vi "GDSII_Parser_Prototype.vi"() -> ()   [LabVIEW 2019]
uses:
  2b7293ed-e710-4ec8-a3ce-adb50af5e69b.vi
  1c682564-4fc3-4e5f-8e88-aad9faa58424.vi
  0011f8b4-c6ad-40f6-b327-4618c1387816.vi
  5f04ecbc-5114-4225-9cf0-5074f08f4171.vi
  <vilib>/JDP Science/JSONtext/Variant to JSON Text.vi
  <vilib>/JDP Science/JSONtext/LVClass Serializer/JSONtext LVClass Serializer.lvclass
panel:
  in  "Path":path=path "C:/Users/Albro/Downloads/Aditi_GDSII/Aditi_GDSII.gds"
  out "Record Str":string
  out "Record Values":string[](array[string])
  out "Record Types Array":string[](array[string])
  # "[\n    2021,\n    1,\n    24,\n    20,\n    0,\n    15,\n    2021,\n    1,\n    24,\n    20,\n    0,\n    15\n]"
  # "[\n    8.16583633422852E-9,\n    7.98085213557943E-33\n]"
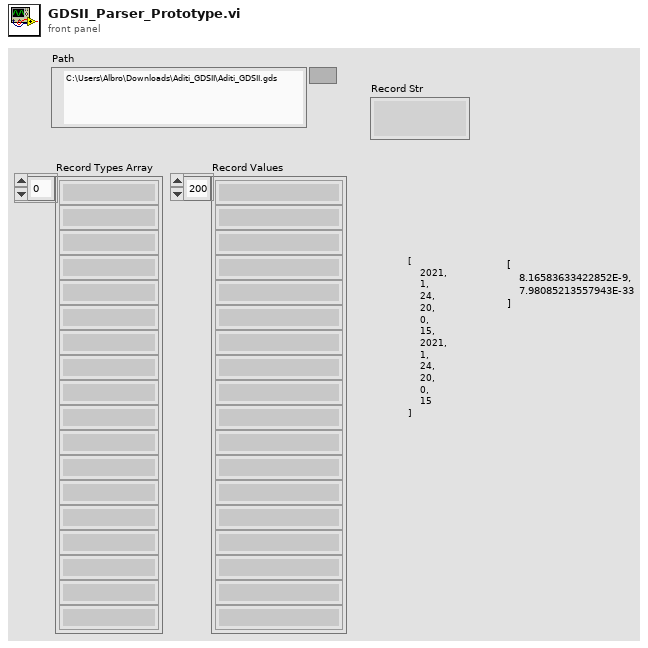
[diagram p1: front panel]
types:
  T1 = enum32{"Invalid", "Standard", "Closed", "Hidden", "Minimized", "Maximized"}
  T2 = enum32{"invalid app kind", "Development System", "Run Time System", "Student Edition", "Embedded LabVIEW", "Evaluation", "Custom"}
  T3 = cluster{"Core":cluster{"Current VI Reference":refnum<vi>, "Close Panel on Exit?":bool}, "Raw Str":string, "Record Str":string, "Records":string[], "Record Index":i32, "Record Type":i16, "Record Types Array":string[], "Record Values":string[]}
  T4 = cluster{"Current VI Reference":refnum<vi>, "Close Panel on Exit?":bool}
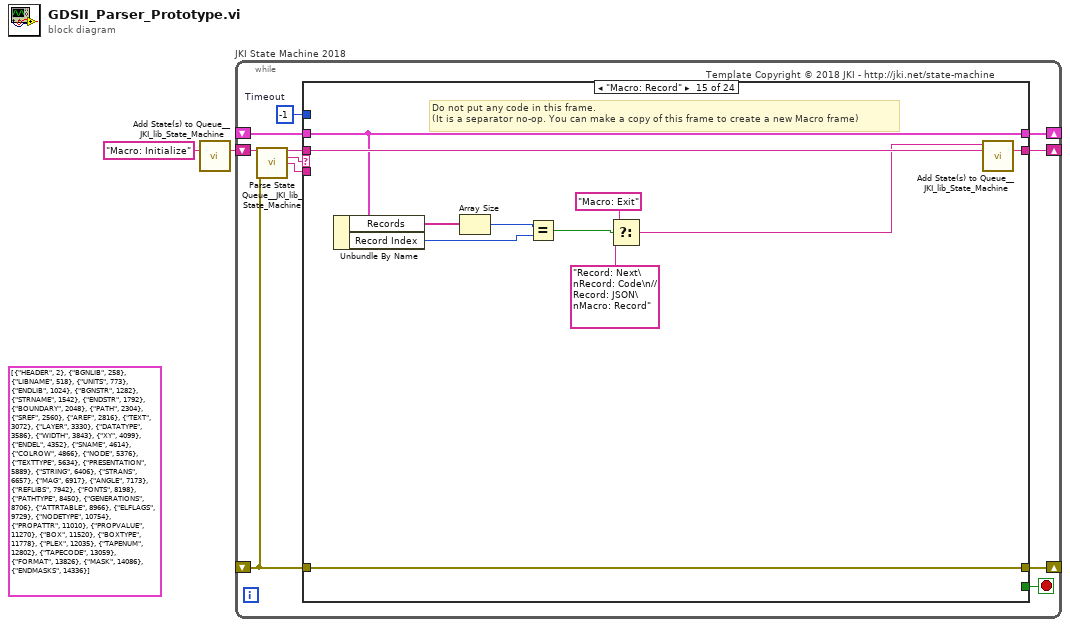
[diagram p0: block diagram]
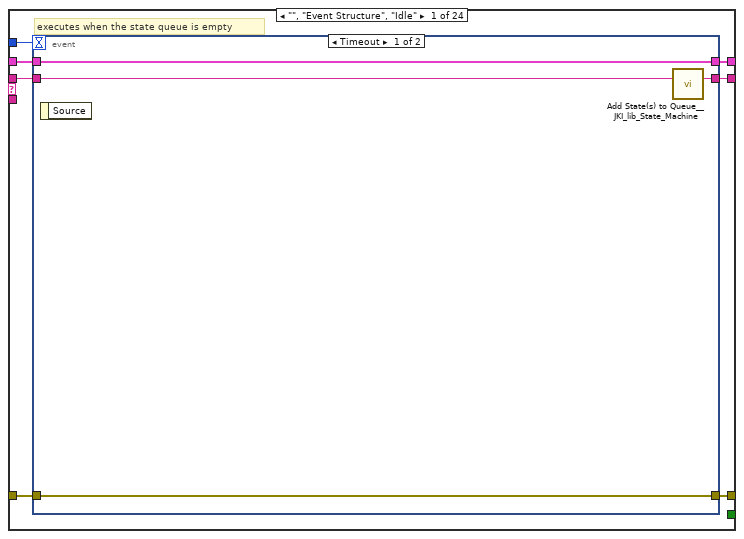
[diagram p2: hidden frame]
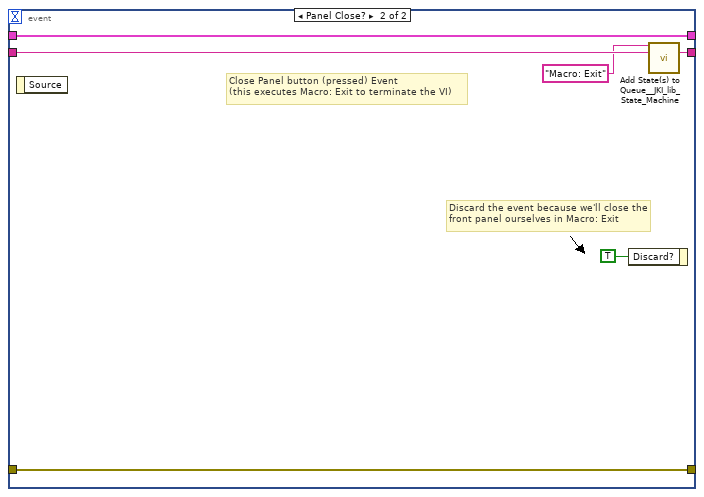
[diagram p3: hidden frame]
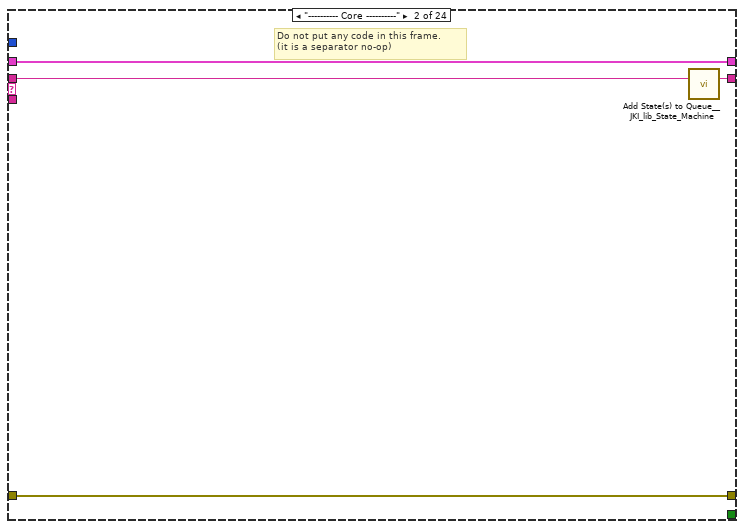
[diagram p4: hidden frame]
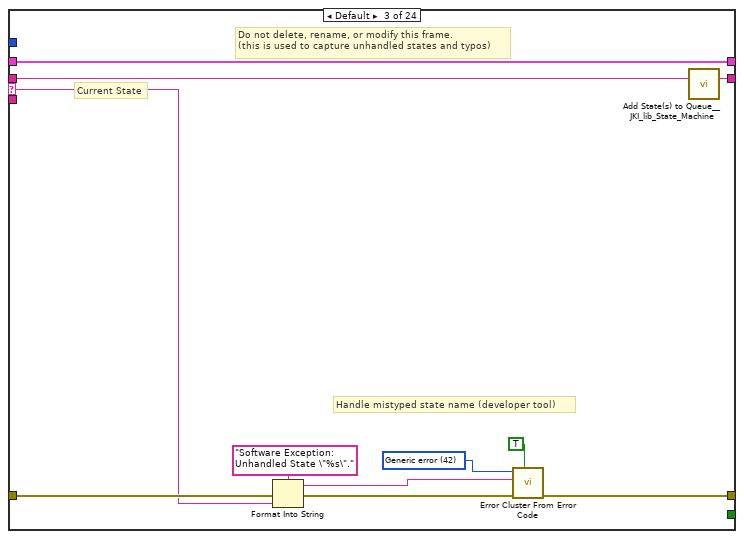
[diagram p5: hidden frame]
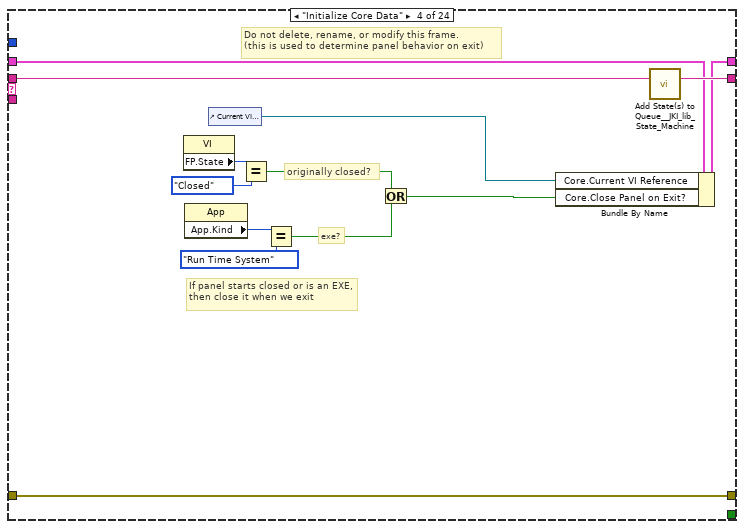
[diagram p6: hidden frame]
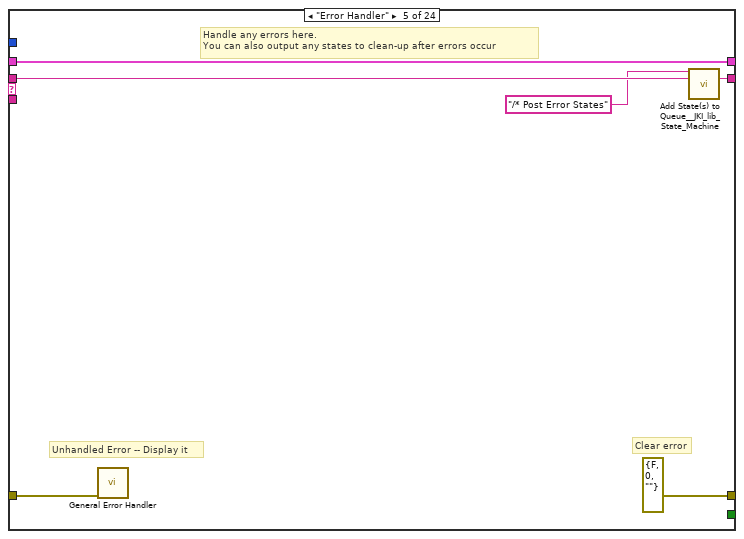
[diagram p7: hidden frame]
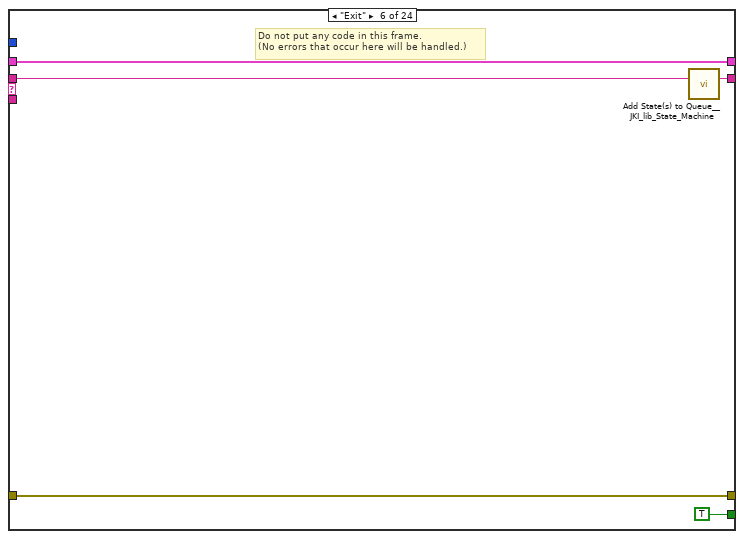
[diagram p8: hidden frame]
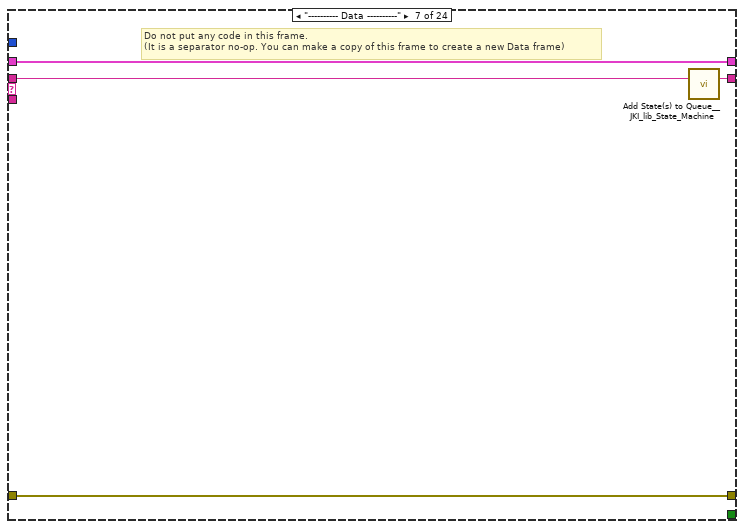
[diagram p9: hidden frame]
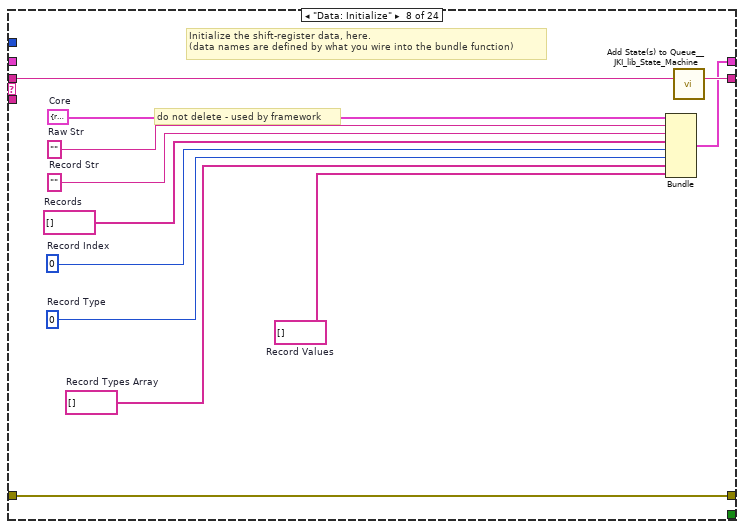
[diagram p10: hidden frame]
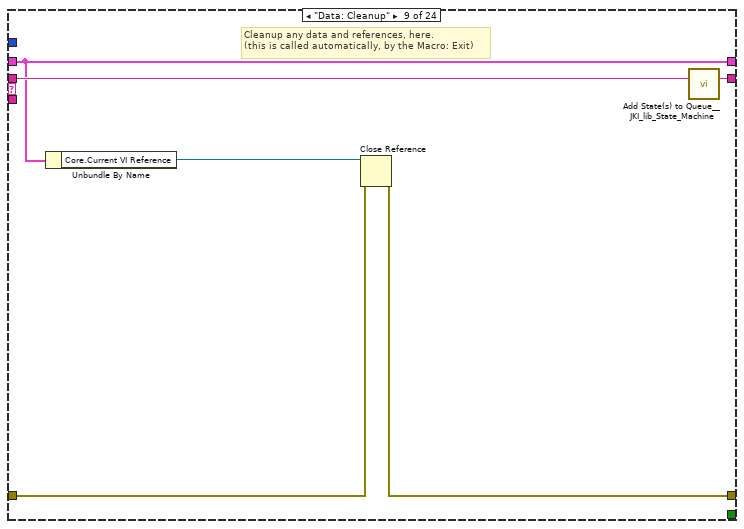
[diagram p11: hidden frame]
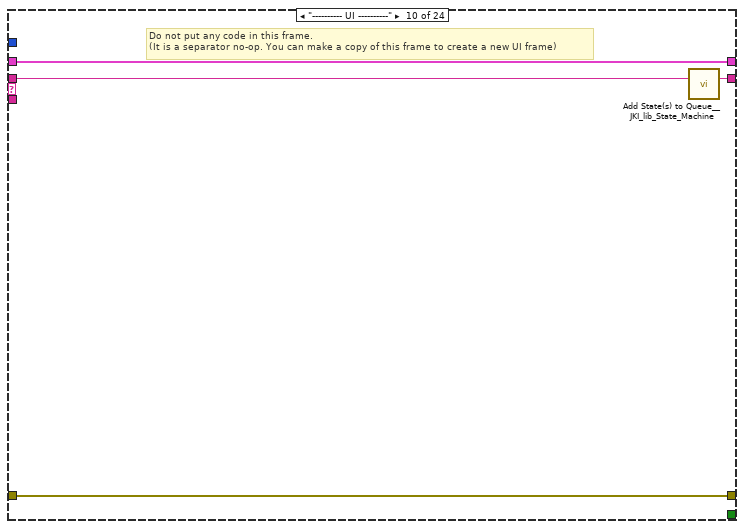
[diagram p12: hidden frame]
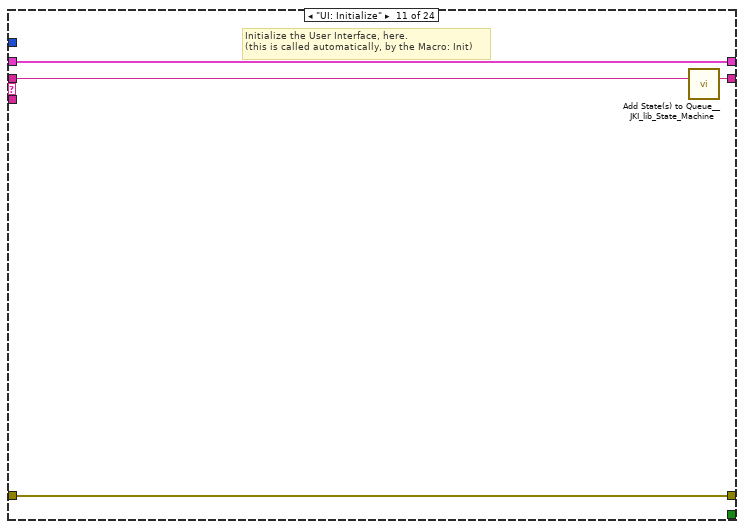
[diagram p13: hidden frame]
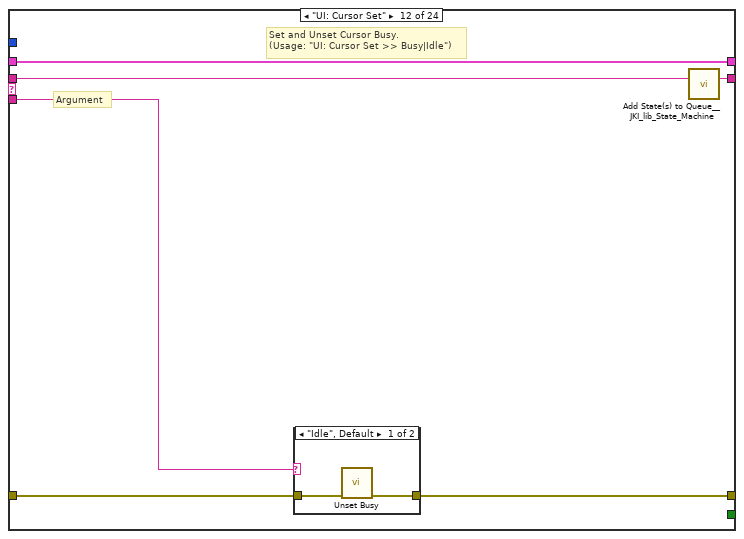
[diagram p14: hidden frame]
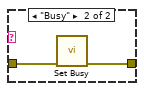
[diagram p15: hidden frame]
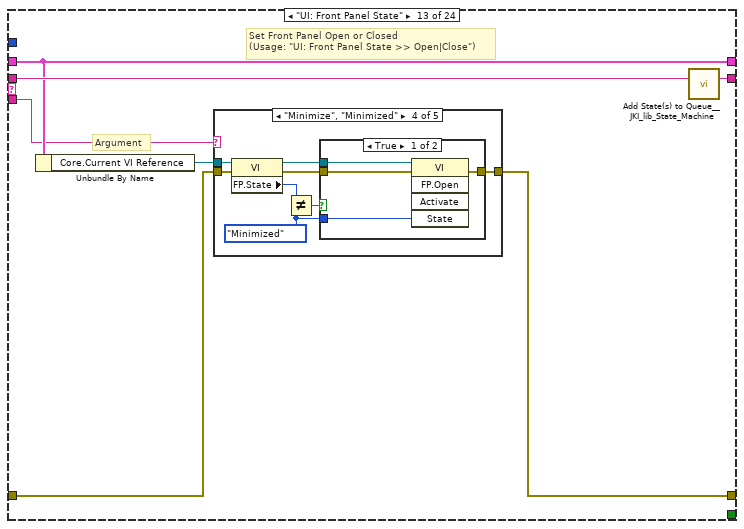
[diagram p16: hidden frame]
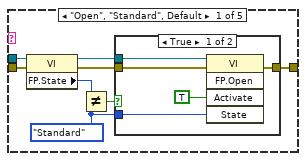
[diagram p17: hidden frame]
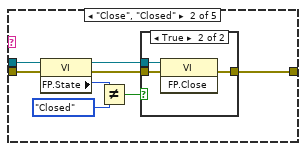
[diagram p19: hidden frame]
diagram:
  (unwired) cluster{"Mnemonic":string, "Code":i16}[] [{"Mnemonic"="HEADER", "Code"=2}, {"Mnemonic"="BGNLIB", "Code"=258}, {"Mnemonic"="LIBNAME", "Code"=518}, {"Mnemonic"="UNITS", "Code"=773}, {"Mnemonic"="ENDLIB", "Code"=1024}, {"Mnemonic"="BGNSTR", "Code"=1282}, {"Mnemonic"="STRNAME", "Code"=1542}, {"Mnemonic"="ENDSTR", "Code"=1792}, {"Mnemonic"="BOUNDARY", "Code"=2048}, {"Mnemonic"="PATH", "Code"=2304}, {"Mnemonic"="SREF", "Code"=2560}, {"Mnemonic"="AREF", "Code"=2816}, {"Mnemonic"="TEXT", "Code"=3072}, {"Mnemonic"="LAYER", "Code"=3330}, {"Mnemonic"="DATATYPE", "Code"=3586}, {"Mnemonic"="WIDTH", "Code"=3843}, {"Mnemonic"="XY", "Code"=4099}, {"Mnemonic"="ENDEL", "Code"=4352}, {"Mnemonic"="SNAME", "Code"=4614}, {"Mnemonic"="COLROW", "Code"=4866}, {"Mnemonic"="NODE", "Code"=5376}, {"Mnemonic"="TEXTTYPE", "Code"=5634}, {"Mnemonic"="PRESENTATION", "Code"=5889}, {"Mnemonic"="STRING", "Code"=6406}, {"Mnemonic"="STRANS", "Code"=6657}, {"Mnemonic"="MAG", "Code"=6917}, {"Mnemonic"="ANGLE", "Code"=7173}, {"Mnemonic"="REFLIBS", "Code"=7942}, {"Mnemonic"="FONTS", "Code"=8198}, {"Mnemonic"="PATHTYPE", "Code"=8450}, {"Mnemonic"="GENERATIONS", "Code"=8706}, {"Mnemonic"="ATTRTABLE", "Code"=8966}, {"Mnemonic"="ELFLAGS", "Code"=9729}, {"Mnemonic"="NODETYPE", "Code"=10754}, {"Mnemonic"="PROPATTR", "Code"=11010}, {"Mnemonic"="PROPVALUE", "Code"=11270}, {"Mnemonic"="BOX", "Code"=11520}, {"Mnemonic"="BOXTYPE", "Code"=11778}, {"Mnemonic"="PLEX", "Code"=12035}, {"Mnemonic"="TAPENUM", "Code"=12802}, {"Mnemonic"="TAPECODE", "Code"=13059}, {"Mnemonic"="FORMAT", "Code"=13826}, {"Mnemonic"="MASK", "Code"=14086}, {"Mnemonic"="ENDMASKS", "Code"=14336}] ("Record Types")
  n1 = call <vilib>:"Add State(s) to Queue__JKI_lib_State_Machine.vi"("State(s) in (\"\")"="Macro: Initialize") -> ("States Out"=w2:string)  [unwired: 14 in]
  n2 = while "JKI State Machine 2018" {
    shift-right: [w6] -> _
    shift-left: _ -> [w5]
    shift-right: [w9] -> _
    shift-left: _ -> [w3]
    shift-right: [w8] -> _
    shift-left: w2 -> [w10]
    stop <- w7 stop-if-true
    w4 = -1  # Timeout
    # "Template Copyright © 2018 JKI - http://jki.net/state-machine"
    n3 = call <vilib>:"Parse State Queue__JKI_lib_State_Machine.vi"("State Queue"=w10, "Error In (no error)"=w3) -> ("Remaining States"=w12:string, "Current State"=w13:string, "Arguments"=w11:string)  [unwired: 11 in]
    n4 = case shown="\"Macro: Record\"" w13 {
      selector: w13 -> [_ _ w35 _ _ _ _ _ _ _ _ _ _ _ _ _ _ _ _ _ _ _ _ _]
      tunnel: w12 -> [w20 w34 w39 w58 w64 w69 w73 w85 w91 w95 w99 w105 w116 w185 w196 w201 w213 w217 w229 w239 w255 w267 w315 w324]
      tunnel: w11 -> [_ _ _ _ _ _ _ _ _ _ _ w100 w110 _ _ _ _ _ _ _ _ _ _ _]
      tunnel: w5 -> [w18 w31 w37 w51 w61 w67 w70 _ w86 w92 w97 w103 w112 w182 w193 w198 w210 w214 w220 w231 w251 w263 w311 w320]
      tunnel: [w17 w32 w41 w55 errorcluster {"status"=FALSE, "code"=0, "source"=""} ("error out") w66 w71 w82 w87 w93 w96 w101 w113 w183 w194 w199 w211 w215 w223 w237 w253 w265 w313 w322] -> w9
      tunnel: w3 -> [w16 w32 w40 w55 w60 w66 w71 w82 w88 w93 w96 w102 w114 w183 w194 w199 w211 w215 w222 w237 w253 w265 w313 w322]
      tunnel: [w19 w33 w38 w57 w63 w68 w72 w84 w90 w94 w98 w104 w115 w184 w195 w200 w212 w216 w228 w238 w254 w266 w314 w323] -> w8
      tunnel: [_ _ _ _ _ TRUE _ _ _ _ _ _ _ _ _ _ _ _ _ _ _ _ _ _] -> w7
      tunnel: [w15 w31 w37 w56 w61 w67 w70 w83 w86 w92 w97 w103 w112 w182 w193 w198 w210 w214 w221 w232 w252 w264 w312 w321] -> w6
      tunnel: w4 -> [w14 _ _ _ _ _ _ _ _ _ _ _ _ _ _ _ _ _ _ _ _ _ _ _]
      frame "", "Event Structure", "Idle" {
        # "executes when the state queue is empty"
        n5 = event shown="[0] Timeout" {
          selector: _ -> [_ _]
          dyn-events: _ -> [_ _]
          timeout: w14 -> [_ _]
          tunnel: w20 -> [w24 w30]
          tunnel: [w23 w29] -> w19
          tunnel: w18 -> [w21 w27]
          tunnel: [w22 w28] -> w17
          tunnel: w16 -> [w22 w28]
          tunnel: [w21 w27] -> w15
          event Timeout {
            n6 = event-data() -> ()  [unwired: 1 in, 1 out]
            n7 = call <vilib>:"Add State(s) to Queue__JKI_lib_State_Machine.vi"("State(s) in (\"\")"=w24) -> ("States Out"=w23:string)  [unwired: 14 in]
          }
          event Panel Close? {
            # "Discard the event because we'll close the front panel ourselves in Macro: Exit"
            # "Close Panel button (pressed) Event\n(this executes Macro: Exit to terminate the VI)"
            n8 = event-data() -> ()  [unwired: 1 in, 1 out]
            n9 = event-data("Discard?"=TRUE) -> ()  [unwired: 1 in, 1 out]
            n10 = call <vilib>:"Add State(s) to Queue__JKI_lib_State_Machine.vi"("State(s) in Front (\"\")"="Macro: Exit", "State(s) in (\"\")"=w30) -> ("States Out"=w29:string)  [unwired: 13 in]
          }
        }
      }
      frame "---------- Core ----------" {
        # "Do not put any code in this frame.\n(it is a separator no-op)"
        n11 = call <vilib>:"Add State(s) to Queue__JKI_lib_State_Machine.vi"("State(s) in (\"\")"=w34) -> ("States Out"=w33:string)  [unwired: 14 in]
      }
      frame Default {
        w44 = 42 items=["No error", "Argument error", "Memory is full", "Out of zone", "End of file", "File already open", "Generic file I/O error", "File not found", "File permission error", "Disk is full", "Duplicate path", "Too many files open", "System feature not enabled", "Resource file not found", "Cannot add resource", "Resource not found", "Image not found", "Image memory error", "Pen does not exist", "Config type invalid", "Config token not found", "Config parse error", "Config memory error", "Bad external code format", "Bad external code offset", "External code not present", "Null window", "Destroy window error", "Null menu", "Print aborted", "Bad print record", "Print driver error", "Windows error during printing", "Memory error during printing", "Print dialog error", "Generic print error", "Invalid device refnum", "Device not found", "Device parameter error", "Device unit error", "Cannot open device", "Device call aborted", "Generic error", "Cancelled by user", "Object ID too low", "Object ID too high", "Object not in heap", "Unknown heap", "Unknown object (invalid DefProc)", "Unknown object (DefProc not in table)", "Message out of range", "Invalid (null) method", "Unknown message", "Manager call not supported", "Bad address", "Network operation in progress", "Network operation timed out", "Connection is busy", "Network attribute not supported", "Network error", "Address in use", "System out of memory", "Connection aborted", "Connection refused", "Not connected", "Already connected", "Connection closed", "Initialization error (interapplication manager)", "Bad occurrence", "Wait on unbound occurrence handler", "Occurrence queue overflow", "Datalog type conflict", "Unused", "Unrecognized type (interapplication manager)", "Memory corrupt", "Failed to make temporary DLL", "Old CIN version", "Drag socket not found", "Failed to load drop-object", "Failed to register OLE object", "Failed to release OLE object", "Format specifier type mismatch", "Unknown format specifier", "Too few format specifiers", "Too many format specifiers", "Scan failed", "Newer CIN version", "Error converting to variant", "Runtime menu error", "Password tampered", "Variant attribute not found", "Incompatible variant data type", "Event data is not available", "Event Store is not present", "Occurrence is not found", "Event Queue is not created", "Event info is not available", "Refnum passed is NULL", "Error retrieving Class GUID", "Error retrieving CoClass GUID", "Error retrieving TypeLib GUID.", "Bad built application magic bytes.", "Specific driver is different from the specific driver associated with the Logical Name.", "There is no session opened to the class driver.", "Max Error", "MAX - Error with config objects", "MAX - Error loading configuration", "MAX - Group not supported"]
        # "Current State"
        # "Do not delete, rename, or modify this frame.\n(this is used to capture unhandled states and typos)"
        # "Handle mistyped state name (developer tool)"
        n12 = Format Into String(format string="Software Exception: Unhandled State \"%s\"." ("message"), error in=w40, w35) -> (resulting string=w43:string, error out=w42:errorcluster)  [unwired: 1 in]
        n13 = call <vilib>:"Error Cluster From Error Code.vi"("show call chain? (False)"=TRUE, "error in (no error)"=w42, "error message (\"\")"=w43, "error code (0)"=w44) -> ("error out"=w41:errorcluster)  [unwired: 5 in]
        n14 = call <vilib>:"Add State(s) to Queue__JKI_lib_State_Machine.vi"("State(s) in (\"\")"=w39) -> ("States Out"=w38:string)  [unwired: 14 in]
      }
      frame "Initialize Core Data" {
        # "Do not delete, rename, or modify this frame.\n(this is used to determine panel behavior on exit)"
        # "originally closed?"
        # "exe?"
        # "If panel starts closed or is an EXE, then close it when we exit"
        n15 = property class="VI"() -> ("FP.State"=w48:T1)  [unwired: 2 in, 2 out]
        n16 = property class="App"() -> ("App.Kind"=w54:T2)  [unwired: 2 in, 2 out]
        n17 = control-ref of="Current VI Reference"() -> (w49:refnum<vi>)
        n18 = Equal?(x=w48, y=T1."Closed" ("Front Panel Window:State")) -> (x = y?=w46:bool)
        n19 = Equal?(x=w54, y=T2."Run Time System" ("Application:Kind")) -> (x = y?=w52:bool)
        n20 = Or(x=w46, y=w52) -> (x .or. y?=w50:bool)
        n21 = Bundle By Name(cluster=w51, "Core.Current VI Reference"=w49, "Core.Close Panel on Exit?"=w50) -> (w56:T3)
        n22 = call <vilib>:"Add State(s) to Queue__JKI_lib_State_Machine.vi"("State(s) in (\"\")"=w58) -> ("States Out"=w57:string)  [unwired: 14 in]
      }
      frame "Error Handler" {
        # "Unhandled Error -- Display it"
        # "Handle any errors here.\nYou can also output any states to clean-up after errors occur"
        # "Clear error"
        n23 = call <vilib>:"General Error Handler.vi"("error in (no error)"=w60) -> ()  [unwired: 10 in, 5 out]
        n24 = call <vilib>:"Add State(s) to Queue__JKI_lib_State_Machine.vi"("State(s) in Front (\"\")"="/* Post Error States", "State(s) in (\"\")"=w64) -> ("States Out"=w63:string)  [unwired: 13 in]
      }
      frame "Exit" {
        # "Do not put any code in this frame.\n(No errors that occur here will be handled.)"
        n25 = call <vilib>:"Add State(s) to Queue__JKI_lib_State_Machine.vi"("State(s) in (\"\")"=w69) -> ("States Out"=w68:string)  [unwired: 14 in]
      }
      frame "---------- Data ----------" {
        # "Do not put any code in this frame.\n(It is a separator no-op. You can make a copy of this frame to create a new Data frame)"
        n26 = call <vilib>:"Add State(s) to Queue__JKI_lib_State_Machine.vi"("State(s) in (\"\")"=w73) -> ("States Out"=w72:string)  [unwired: 14 in]
      }
      frame "Data: Initialize" {
        w74 = string[] []  # Record Values
        w75 = string[] []  # Record Types Array
        w76 = i16 0  # Record Type
        w77 = 0  # Record Index
        w78 = ""  # Raw Str
        w79 = string[] []  # Records
        w81 = T4 {"Current VI Reference"=refnum, "Close Panel on Exit?"=FALSE}  # Core
        w80 = ""  # Record Str
        # "do not delete - used by framework"
        # "Initialize the shift-register data, here.\n(data names are defined by what you wire into the bundle function)"
        n27 = Bundle("Core"=w81, "Raw Str"=w78, "Record Str"=w80, "Records"=w79, "Record Index"=w77, "Record Type"=w76, "Record Types Array"=w75, "Record Values"=w74) -> (w83:T3)  [unwired: 1 in]
        n28 = call <vilib>:"Add State(s) to Queue__JKI_lib_State_Machine.vi"("State(s) in (\"\")"=w85) -> ("States Out"=w84:string)  [unwired: 14 in]
      }
      frame "Data: Cleanup" {
        # "Cleanup any data and references, here.\n(this is called automatically, by the Macro: Exit)"
        n29 = Unbundle By Name(w86) -> ("Core.Current VI Reference"=w89:refnum<vi>)
        n30 = Close Reference(reference=w89, error in (no error)=w88) -> (error out=w87:errorcluster)
        n31 = call <vilib>:"Add State(s) to Queue__JKI_lib_State_Machine.vi"("State(s) in (\"\")"=w91) -> ("States Out"=w90:string)  [unwired: 14 in]
      }
      frame "---------- UI ----------" {
        # "Do not put any code in this frame.\n(It is a separator no-op. You can make a copy of this frame to create a new UI frame)"
        n32 = call <vilib>:"Add State(s) to Queue__JKI_lib_State_Machine.vi"("State(s) in (\"\")"=w95) -> ("States Out"=w94:string)  [unwired: 14 in]
      }
      frame "UI: Initialize" {
        # "Initialize the User Interface, here.\n(this is called automatically, by the Macro: Init)"
        n33 = call <vilib>:"Add State(s) to Queue__JKI_lib_State_Machine.vi"("State(s) in (\"\")"=w99) -> ("States Out"=w98:string)  [unwired: 14 in]
      }
      frame "UI: Cursor Set" {
        # "Argument"
        # "Set and Unset Cursor Busy.\n(Usage: \"UI: Cursor Set >> Busy|Idle\")"
        n34 = case shown="\"Idle\", Default" w100 {
          tunnel: w102 -> [w107 w109]
          tunnel: [w106 w108] -> w101
          frame "Idle", Default {
            n35 = call <vilib>:"Unset Busy.vi"("error in (no error)"=w107) -> ("error out"=w106:errorcluster)  [unwired: 10 in]
          }
          frame "Busy" {
            n36 = call <vilib>:"Set Busy.vi"("error in (no error)"=w109) -> ("error out"=w108:errorcluster)  [unwired: 9 in, 1 out]
          }
        }
        n37 = call <vilib>:"Add State(s) to Queue__JKI_lib_State_Machine.vi"("State(s) in (\"\")"=w105) -> ("States Out"=w104:string)  [unwired: 14 in]
      }
      frame "UI: Front Panel State" {
        # "Argument"
        # "Set Front Panel Open or Closed\n(Usage: \"UI: Front Panel State >> Open|Close\")"
        n38 = Unbundle By Name(w112) -> ("Core.Current VI Reference"=w111:refnum<vi>)
        n39 = case shown="\"Minimize\", \"Minimized\"" w110 {
          tunnel: w114 -> [w122 w137 w148 w161 w174]
          tunnel: [w124 w138 w150 w163 w176] -> w113
          tunnel: w111 -> [w123 w135 w149 w162 w175]
          frame "Open", "Standard", Default {
            w117 = T1."Standard" ("State")
            n40 = property class="VI"(reference=w123, error in=w122) -> (reference out=w120:refnum<vi>, error out=w121:errorcluster, "FP.State"=w119:T1)
            n41 = Not Equal?(x=w119, y=w117) -> (x != y?=w118:bool)
            n42 = case shown="True" w118 {
              tunnel: [w128 w130] -> w124
              tunnel: w121 -> [w127 w130]
              tunnel: w120 -> [w126 _]
              tunnel: w117 -> [w125 _]
              frame True {
                n43 = invoke class="VI" method="FP.Open"(reference=w126, error in=w127, "Activate"=TRUE, "State"=w125) -> (error out=w128:errorcluster)  [unwired: 1 in, 4 out]
              }
              frame False {
              }
            }
          }
          frame "Close", "Closed" {
            n44 = property class="VI"(reference=w135, error in=w137) -> (reference out=w134:refnum<vi>, error out=w136:errorcluster, "FP.State"=w132:T1)
            n45 = Not Equal?(x=w132, y=T1."Closed" ("Front Panel Window:State")) -> (x != y?=w131:bool)
            n46 = case shown="True" w131 {
              tunnel: [w139 w142] -> w138
              tunnel: w136 -> [w139 w141]
              tunnel: w134 -> [_ w140]
              frame False {
              }
              frame True {
                n47 = invoke class="VI" method="FP.Close"(reference=w140, error in=w141) -> (error out=w142:errorcluster)  [unwired: 1 in, 2 out]
              }
            }
          }
          frame "Hidden", "Hide" {
            w143 = T1."Hidden" ("State")
            n48 = property class="VI"(reference=w149, error in=w148) -> (reference out=w146:refnum<vi>, error out=w147:errorcluster, "FP.State"=w145:T1)
            n49 = Not Equal?(x=w145, y=w143) -> (x != y?=w144:bool)
            n50 = case shown="True" w144 {
              tunnel: [w154 w155] -> w150
              tunnel: w147 -> [w153 w155]
              tunnel: w146 -> [w152 _]
              tunnel: w143 -> [w151 _]
              frame True {
                n51 = invoke class="VI" method="FP.Open"(reference=w152, error in=w153, "State"=w151) -> (error out=w154:errorcluster)  [unwired: 2 in, 4 out]
              }
              frame False {
              }
            }
          }
          frame "Minimize", "Minimized" {
            w156 = T1."Minimized" ("State")
            n52 = property class="VI"(reference=w162, error in=w161) -> (reference out=w159:refnum<vi>, error out=w160:errorcluster, "FP.State"=w158:T1)
            n53 = Not Equal?(x=w158, y=w156) -> (x != y?=w157:bool)
            n54 = case shown="True" w157 {
              tunnel: [w167 w168] -> w163
              tunnel: w160 -> [w166 w168]
              tunnel: w159 -> [w165 _]
              tunnel: w156 -> [w164 _]
              frame True {
                n55 = invoke class="VI" method="FP.Open"(reference=w165, error in=w166, "State"=w164) -> (error out=w167:errorcluster)  [unwired: 2 in, 4 out]
              }
              frame False {
              }
            }
          }
          frame "Maximize", "Maximized" {
            w169 = T1."Maximized" ("State")
            n56 = property class="VI"(reference=w175, error in=w174) -> (reference out=w172:refnum<vi>, error out=w173:errorcluster, "FP.State"=w171:T1)
            n57 = Not Equal?(x=w171, y=w169) -> (x != y?=w170:bool)
            n58 = case shown="True" w170 {
              tunnel: [w180 w181] -> w176
              tunnel: w173 -> [w179 w181]
              tunnel: w172 -> [w178 _]
              tunnel: w169 -> [w177 _]
              frame True {
                n59 = invoke class="VI" method="FP.Open"(reference=w178, error in=w179, "State"=w177) -> (error out=w180:errorcluster)  [unwired: 2 in, 4 out]
              }
              frame False {
              }
            }
          }
        }
        n60 = call <vilib>:"Add State(s) to Queue__JKI_lib_State_Machine.vi"("State(s) in (\"\")"=w116) -> ("States Out"=w115:string)  [unwired: 14 in]
      }
      frame "---------- Macro ----------" {
        # "Do not put any code in this frame.\n(It is a separator no-op. You can make a copy of this frame to create a new Macro frame)"
        n61 = call <vilib>:"Add State(s) to Queue__JKI_lib_State_Machine.vi"("State(s) in (\"\")"=w185) -> ("States Out"=w184:string)  [unwired: 14 in]
      }
      frame "Macro: Record" {
        # "Do not put any code in this frame.\n(It is a separator no-op. You can make a copy of this frame to create a new Macro frame)"
        n62 = Unbundle By Name(w193) -> ("Records"=w192:string[], "Record Index"=w190:i32)
        n63 = Array Size(array=w192) -> (size(s)=w191:i32)
        n64 = Equal?(x=w191, y=w190) -> (x = y?=w189:bool)
        n65 = Select(t="Macro: Exit", s=w189, f="Record: Next\nRecord: Code\n//Record: JSON\nMacro: Record") -> (s? t:f=w186:string)
        n66 = call <vilib>:"Add State(s) to Queue__JKI_lib_State_Machine.vi"("State(s) in Front (\"\")"=w186, "State(s) in (\"\")"=w196) -> ("States Out"=w195:string)  [unwired: 13 in]
      }
      frame "Macro: Initialize" {
        # "Initialization Macro\n(This is called once, when the VI starts)"
        n67 = call <vilib>:"Add State(s) to Queue__JKI_lib_State_Machine.vi"("State(s) in Front (\"\")"="Data: Initialize\nInitialize Core Data\nUI: Initialize\nUI: Front Panel State >> Open\nFile: Read\nFile: Split\nRecord: Next\nRecord: Code\nRecord: JSON\nRecord: Next\nRecord: Code\nRecord: JSON\nRecord: Next\nRecord: Code\nRecord: JSON\nMacro: Record", "State(s) in (\"\")"=w201) -> ("States Out"=w200:string)  [unwired: 13 in]
      }
      frame "Macro: Exit" {
        # "Exit Macro\n(This is called once, when the VI exits)"
        n68 = Unbundle By Name(w210) -> ("Core.Close Panel on Exit?"=w209:bool, "Record Types Array"=→"Record Types Array":string[], "Record Values"=→"Record Values":string[])
        n69 = Select(t="UI: Front Panel State >> Close", s=w209, f="") -> (s? t:f=w206:string)
        n70 = call <vilib>:"Add State(s) to Queue__JKI_lib_State_Machine.vi"("State(s) in (\"\")"=w206, "State(s) at Back (\"\")"="Data: Cleanup\nExit") -> ("States Out"=w204:string)  [unwired: 13 in]
        n71 = call <vilib>:"Add State(s) to Queue__JKI_lib_State_Machine.vi"("State(s) in Front (\"\")"=w204, "State(s) in (\"\")"=w213) -> ("States Out"=w212:string)  [unwired: 13 in]
      }
      frame "---------- File ----------" {
        # "Template Separator\n(You can make a copy of, or modify, this frame)"
        n72 = call <vilib>:"Add State(s) to Queue__JKI_lib_State_Machine.vi"("State(s) in (\"\")"=w217) -> ("States Out"=w216:string)  [unwired: 14 in]
      }
      frame "File: Read" {
        # "Your code here.\n(You can make a copy of, or modify, this frame)"
        n73 = Open/Create/Replace File(file path (use dialog)="Path", error in=w222) -> (refnum out=w227:refnum<file>, error out=w225:errorcluster)  [unwired: 4 in, 1 out]
        n74 = Read from Text File(file (use dialog)=w227, error in=w225) -> (refnum out=w226:refnum<file>, text=w219:string, error out=w224:errorcluster)  [unwired: 2 in, 1 out]
        n75 = Bundle By Name(cluster=w220, "Raw Str"=w219) -> (w221:T3)
        n76 = Close File(refnum=w226, error in=w224) -> (error out=w223:errorcluster)  [unwired: 1 out]
        n77 = call <vilib>:"Add State(s) to Queue__JKI_lib_State_Machine.vi"("State(s) in (\"\")"=w229) -> ("States Out"=w228:string)  [unwired: 14 in]
      }
      frame "File: Split" {
        # "Template Separator\n(You can make a copy of, or modify, this frame)"
        n78 = Unbundle By Name(w231) -> ("Raw Str"=w234:string)
        n79 = String Length(string=w234) -> (length=w235:i32)
        n80 = Decrement(x=w235) -> (x-1=w233:i32)
        n81 = while {
          tunnel: w234 -> [w244]
          shift-right: [w241] -> _
          shift-left: 0 -> [w243]
          tunnel: w233 -> [w248]
          tunnel: [w240] -> w230 mode=indexing
          stop <- w249 stop-if-true
          n82 = Greater Or Equal?(x=w243, y=w248) -> (x >= y?=w249:bool)
          n83 = String Subset(string=w244, offset (0)=w243, length (rest)=2 ("length (rest)")) -> (substring=w246:string)
          n84 = Type Cast(type=i16 0, x=w246) -> (*(type *) &x=w242:i16)
          n85 = String Subset(string=w244, offset (0)=w243, length (rest)=w242) -> (substring=w240:string)
          n86 = Add(x=w243, y=w242) -> (x+y=w241:i32)
        }
        n87 = Bundle By Name(cluster=w231, "Records"=w230) -> (w232:T3)
        n88 = call <vilib>:"Add State(s) to Queue__JKI_lib_State_Machine.vi"("State(s) in (\"\")"=w239) -> ("States Out"=w238:string)  [unwired: 14 in]
      }
      frame "---------- Record ----------" {
        # "Template Separator\n(You can make a copy of, or modify, this frame)"
        n89 = Unbundle By Name(w251) -> ("Record Str"=w250:string)
        n90 = Bundle By Name(cluster=w251, "Record Str"=w250) -> (w252:T3)
        n91 = call <vilib>:"Add State(s) to Queue__JKI_lib_State_Machine.vi"("State(s) in (\"\")"=w255) -> ("States Out"=w254:string)  [unwired: 14 in]
      }
      frame "Record: JSON" {
        # "Template Separator\n(You can make a copy of, or modify, this frame)"
        n92 = Unbundle By Name(w263) -> ("Record Values"=w258:string[], "Record Str"=w261:string, "Record Type"=w262:i16)
        n93 = String Subset(string=w261, offset (0)=4) -> (substring=w259:string)  [unwired: 1 in]
        n94 = case shown="2" w262 {
          tunnel: w259 -> [_ w272 w280 w285 w293 _]
          tunnel: ["" w269 w278 w286 w295 ""] -> w257
          frame Default {
          }
          frame 2 {
            n95 = Type Cast(type=i16 0, x=w272) -> (*(type *) &x=w270:i16)
            n96 = disable-structure shown="Enabled" {
              disable-tunnel: w270 -> [w274 w275]
              disable-tunnel: [w273 w276] -> w269
              frame Disabled {
                n97 = call <vilib>:"Flatten To JSON String.vi"("Variant"=w274) -> ("JSON String"=w273:string)  [unwired: 9 in, 1 out]
              }
              frame Enabled {
                n98 = call "To JSON Text.vim"("Anything"=w275) -> ("<JSON>"=w276:string)  [unwired: 9 in, 1 out]
              }
            }
          }
          frame 258 {
            n99 = Type Cast(type=i16[] [], x=w280) -> (*(type *) &x=w279:i16[])
            n100 = disable-structure shown="Enabled" {
              disable-tunnel: w279 -> [w282 w284]
              disable-tunnel: [w281 w283] -> w278
              frame Disabled {
                n101 = call <vilib>:"Flatten To JSON String.vi"("Variant"=w282) -> ("JSON String"=w281:string)  [unwired: 9 in, 1 out]
              }
              frame Enabled {
                n102 = call "To JSON Text.vim"("Anything"=w284) -> ("<JSON>"=w283:string)  [unwired: 9 in, 1 out]
              }
            }
          }
          frame 518 {
            n103 = disable-structure shown="Enabled" {
              disable-tunnel: [w288 w289] -> w286
              disable-tunnel: w285 -> [w287 w290]
              frame Disabled {
                n104 = call <vilib>:"Flatten To JSON String.vi"("Variant"=w287) -> ("JSON String"=w288:string)  [unwired: 9 in, 1 out]
              }
              frame Enabled {
                n105 = call "To JSON Text.vim"("Anything"=w290) -> ("<JSON>"=w289:string)  [unwired: 9 in, 1 out]
              }
            }
          }
          frame 773 {
            # "This isnt right in terms of the 8-byte real"
            n106 = String Subset(string=w293, offset (0)=8) -> (substring=w291:string)  [unwired: 1 in]
            n107 = Type Cast(x=w291) -> (*(type *) &x=w294:string)  [unwired: 1 in]
            n108 = disable-structure shown="Enabled" {
              disable-tunnel: [w297 w298] -> w295
              disable-tunnel: w294 -> [w296 w299]
              frame Disabled {
                n109 = call <vilib>:"Flatten To JSON String.vi"("Variant"=w296) -> ("JSON String"=w297:string)  [unwired: 9 in, 1 out]
              }
              frame Enabled {
                n110 = call "To JSON Text.vim"("Anything"=w299) -> ("<JSON>"=w298:string)  [unwired: 9 in, 1 out]
              }
            }
            "Record Str" <- w293
          }
          frame 1024 {
          }
        }
        n111 = Build Array (concatenate)(w258, w257) -> (w256:string[])
        n112 = Bundle By Name(cluster=w263, "Record Str"=w261, "Record Values"=w256) -> (w264:T3)
        n113 = call <vilib>:"Add State(s) to Queue__JKI_lib_State_Machine.vi"("State(s) in (\"\")"=w267) -> ("States Out"=w266:string)  [unwired: 14 in]
      }
      frame "Record: Code" {
        w305 = map{i16, string} {2="HEADER", 258="BGNLIB", 518="LIBNAME", 773="UNITS", 1024="ENDLIB", 1282="BGNSTR", 1542="STRNAME", 1792="ENDSTR", 2048="BOUNDARY", 2304="PATH", 2560="SREF", 2816="AREF", 3072="TEXT", 3330="LAYER", 3586="DATATYPE", 3843="WIDTH", 4099="XY", 4352="ENDEL", 4614="SNAME", 4866="COLROW", 5376="NODE", 5634="TEXTTYPE", 5889="PRESENTATION", 6406="STRING", 6657="STRANS", 6917="MAG", 7173="ANGLE", 7942="REFLIBS", 8198="FONTS", 8450="PATHTYPE", 8706="GENERATIONS", 8966="ATTRTABLE", 9729="ELFLAGS", 10754="NODETYPE", 11010="PROPATTR", 11270="PROPVALUE", 11520="BOX", 11778="BOXTYPE", 12035="PLEX", 12802="TAPENUM", 13059="TAPECODE", 13826="FORMAT", 14086="MASK", 14336="ENDMASKS"}  # Map
        # "Template Separator\n(You can make a copy of, or modify, this frame)"
        n114 = Unbundle By Name(w311) -> ("Record Str"=w303:string, "Record Types Array"=w302:string[])
        n115 = String Subset(string=w303, offset (0)=2, length (rest)=2 ("length (rest)")) -> (substring=w308:string)
        n116 = Type Cast(type=i16 0, x=w308) -> (*(type *) &x=w304:i16)
        n117 = Look In Map(map=w305, key=w304) -> (value=w301:string)  [unwired: 1 in, 1 out]
        n118 = Build Array (concatenate)(w302, w301) -> (w306:string[])
        n119 = Bundle By Name(cluster=w311, "Record Str"=w303, "Record Type"=w304, "Record Types Array"=w306) -> (w312:T3)
        n120 = call <vilib>:"Add State(s) to Queue__JKI_lib_State_Machine.vi"("State(s) in (\"\")"=w315) -> ("States Out"=w314:string)  [unwired: 14 in]
      }
      frame "Record: Next" {
        # "Increment for next time."
        # "Template Separator\n(You can make a copy of, or modify, this frame)"
        n121 = Unbundle By Name(w320) -> ("Records"=w319:string[], "Record Index"=w316:i32)
        n122 = Index Array(array=w319, index=w316) -> (element=w318:string)
        n123 = Increment(x=w316) -> (x+1=w317:i32)
        n124 = Bundle By Name(cluster=w320, "Record Str"=w318, "Record Index"=w317) -> (w321:T3)
        n125 = call <vilib>:"Add State(s) to Queue__JKI_lib_State_Machine.vi"("State(s) in (\"\")"=w324) -> ("States Out"=w323:string)  [unwired: 14 in]
      }
    }
  }
